vi "_Construct.vi"(8 "error in (no error)":errorcluster, 11 "Parameters":T1) -> (0 "error out":errorcluster, 3 "Dual Screen out":refnum<class "DualScreenV.lvclass">)   [LabVIEW 2020, in "DualScreenV.lvlib" / "DualScreenV.lvclass"]
doc: "Splitter parameters:\nThe position unit depends on the sizing mode:\n- If mode is \"Proportional\" : the position is relative to the pane size, in %\n- Else : the position is in pixels"
uses:
  DualScreenV.lvclass
  D:/Projets/STEP AT/Bahamut/D&Cs/DualScreen/DualScreen/DualScreen.lvclass
  DualScreen/DualScreen/DualScreenParam.ctl
  support/UI_Actor.lvlibp/UI_Actor/UI_Actor.lvclass
  DualScreen/DualScreen/DualScreen.lvclass
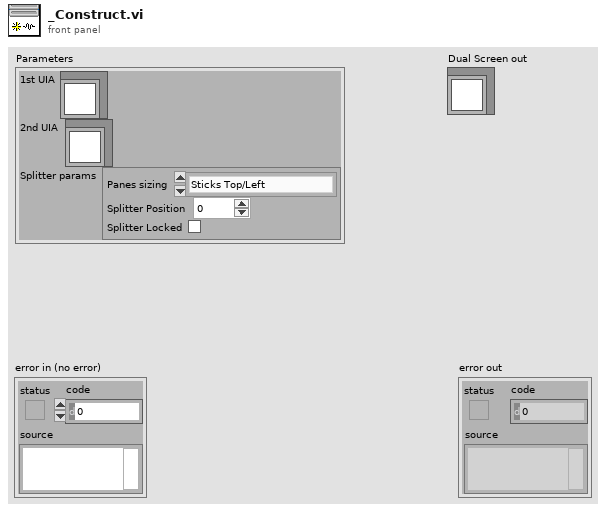
[diagram p1: front panel]
types:
  T1 = typedef "DualScreen.lvlib/DualScreen.lvclass/DualScreenParam.ctl" = cluster{"1st UIA":refnum<class "UI_Actor.lvclass">, "2nd UIA":refnum<class "UI_Actor.lvclass">, "Splitter params":cluster{"Panes sizing":enum16{"Sticks Top/Left", "Sticks Bottom/Right", "Proportional"}, "Splitter Position":i32, "Splitter Locked":bool}}
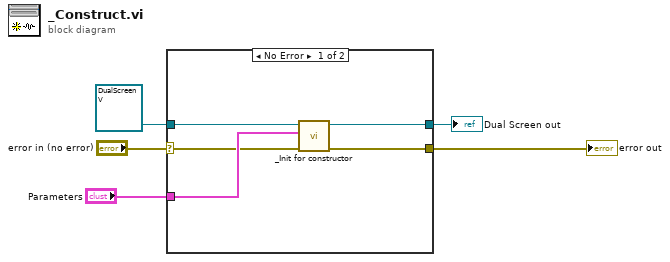
[diagram p0: block diagram]
diagram:
  n1 = case shown="No Error" "error in (no error)" {
    selector: "error in (no error)" -> [w6 w12]
    tunnel: [w8 w12] -> w4
    tunnel: refnum<class "DualScreenV.lvclass"> refnum ("DualScreenV.lvlib:DualScreenV.lvclass") -> [w10 w11]
    tunnel: [w9 w11] -> w3
    tunnel: "Parameters" -> [w7 _]
    frame No Error {
      n2 = call "_Init for constructor.vi"("error in (no error)"=w6, "Parameters"=w7, "DualScreen in"=w10) -> ("error out"=w8:errorcluster, "DualScreen out"=w9:refnum<class "DualScreenV.lvclass">)  [unwired: 7 in]
    }
    frame Error {
    }
  }
  "error out" <- w4
  "Dual Screen out" <- w3
